vi "Modify Error.vi"(8 "error in (no error)":errorcluster, 9 "Append String":string, 10 "Prepend String":string, 11 "Error Code (Original)":i32) -> (0 "error out":errorcluster)   [LabVIEW 2020, in "Volatus.lvlib"]
uses:
  Volatus.lvlib
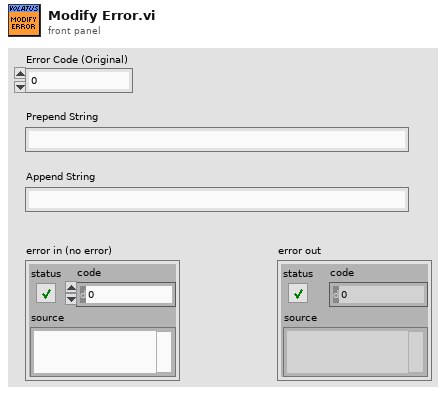
[diagram p1: front panel]
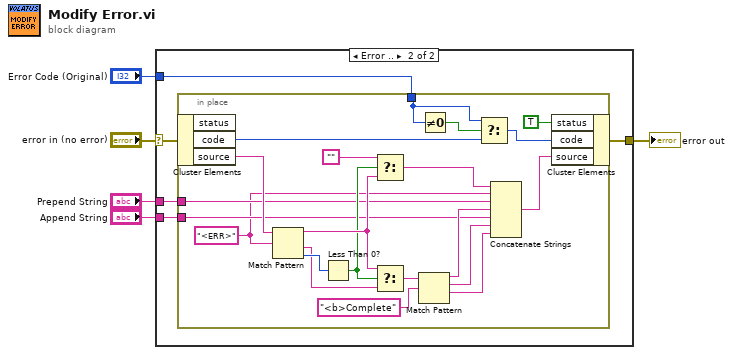
[diagram p0: block diagram]
diagram:
  n1 = case shown="Error .." "error in (no error)" {
    selector: "error in (no error)" -> [w6 w7]
    tunnel: "Error Code (Original)" -> [_ w11]
    tunnel: "Prepend String" -> [_ w10]
    tunnel: "Append String" -> [_ w9]
    tunnel: [w6 w8] -> w2
    frame No Error {
    }
    frame Error {
      n2 = in-place {
        in-place-border: w11 -> [w29]
        in-place-border: w10 -> [w19]
        in-place-border: w9 -> [w17]
        w15 = "<ERR>" ("regular expression")
        n3 = in-place-cluster #1(w7) -> ("code"=w30:i32, "source"=w27:string)  [unwired: 1 out]
        n4 = Match Pattern(string=w27, regular expression=w15) -> (before substring=w22:string, after substring=w25:string, offset past match=w26:i32)  [unwired: 1 in, 1 out]
        n5 = Less Than 0?(x=w26) -> (x < 0?=w21:bool)
        n6 = Select(t="", s=w21, f=w22) -> (s? t:f=w16:string)
        n7 = Select(t=w22, s=w21, f=w25) -> (s? t:f=w24:string)
        n8 = Match Pattern(string=w24, regular expression="<b>Complete") -> (before substring=w18:string, match substring=w14:string, after substring=w13:string)  [unwired: 1 in, 1 out]
        n9 = Not Equal To 0?(x=w29) -> (x != 0?=w28:bool)
        n10 = Select(t=w29, s=w28, f=w30) -> (s? t:f=w31:i32)
        n11 = Concatenate Strings(w16, w15, w19, w18, w17, w14, w13) -> (w12:string)
        n12 = in-place-cluster #1("status"=TRUE, "code"=w31, "source"=w12) -> (w8:errorcluster)
      }
    }
  }
  "error out" <- w2
